vi "Plot load - plots.vi"(8 "error in (no error)":errorcluster, 10 "plots":T2[](array[typedef]), 11 "Refs":T4) -> (0 "error out":errorcluster, 3 "top array.value":T1[](array[typedef]))   [LabVIEW 2021, in "RocketPlot.lvlib"]
uses:
  RocketPlot.lvlib
  TypeDefs/Plot UI references.ctl
  Classes/RocketPlotHandle/RocketPlotHandle.lvclass
  <userlib>/bjustice/TipStripOOPanel/Classes/TipPanelHandle/TipPanelHandle.lvclass
  TypeDefs/Plot top row.ctl
  TypeDefs/plot properties V2.ctl
  TypeDefs/plot attributes V2.ctl
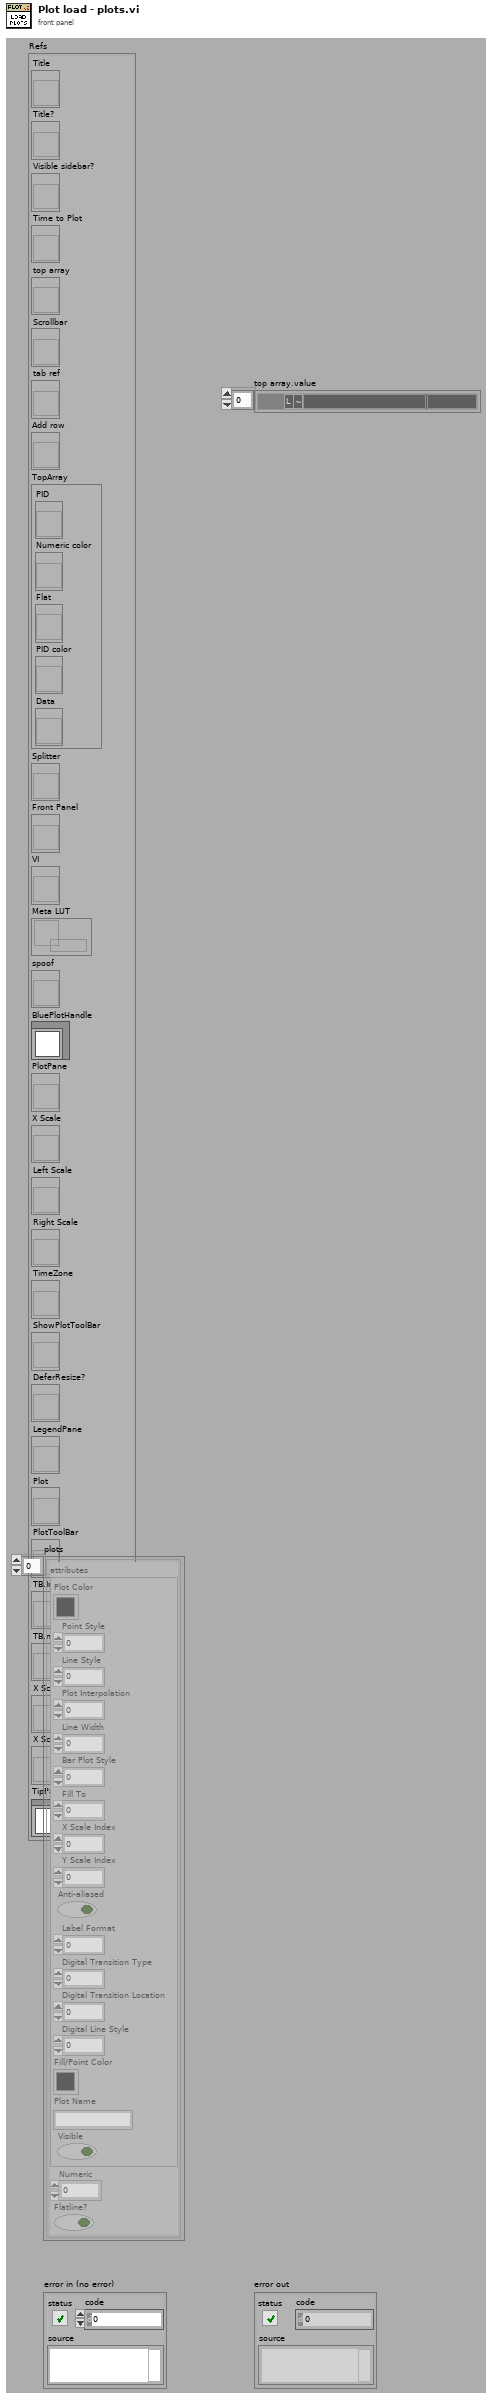
[diagram p1: front panel]
types:
  T1 = typedef "RocketPlot.lvlib/Plot top row.ctl" = cluster{"PID":string, "index":i32, "PID color":u32, "right axis?":bool, "Flatline?":bool, "Numeric color":u32, "Data":string, "Flat":string}
  T2 = typedef "RocketPlot.lvlib/plot properties V2.ctl" = cluster{"attributes":T3, "Numeric":dbl, "Flatline?":bool}
  T3 = typedef "RocketPlot.lvlib/plot attributes V2.ctl" = cluster{"Plot Color":u32, "Point Style":u8, "Line Style":u8, "Plot Interpolation":u8, "Line Width":u8, "Bar Plot Style":u8, "Fill To":i16, "X Scale Index":u32, "Y Scale Index":u32, "Anti-aliased":bool, "Label Format":u8, "Digital Transition Type":u8, "Digital Transition Location":u8, "Digital Line Style":u8, "Fill/Point Color":u32, "Plot Name":string, "Visible":bool}
  T4 = typedef "RocketPlot.lvlib/Plot UI references.ctl" = cluster{"Title":refnum<vi>, "Title?":refnum<vi>, "Visible sidebar?":refnum<vi>, "Time to Plot":refnum<vi>, "top array":refnum<vi>, "Scrollbar":refnum<vi>, "tab ref":refnum<vi>, "Add row":refnum<vi>, "TopArray":cluster{"PID":refnum<vi>, "Numeric color":refnum<vi>, "Flat":refnum<vi>, "PID color":refnum<vi>, "Data":refnum<vi>}, "Splitter":refnum<vi>, "Front Panel":refnum<vi>, "VI":refnum<vi>, "Meta LUT":refnum<data-value>, "spoof":refnum<vi>, "BluePlotHandle":refnum<class "RocketPlotHandle.lvclass">, "PlotPane":refnum<vi>, "X Scale":refnum<vi>, "Left Scale":refnum<vi>, "Right Scale":refnum<vi>, "TimeZone":refnum<vi>, "ShowPlotToolBar":refnum<vi>, "DeferResize?":refnum<vi>, "LegendPane":refnum<vi>, "Plot":refnum<vi>, "PlotToolBar":refnum<vi>, "TB.Info":refnum<vi>, "TB.max":refnum<vi>, "X Scale.Plot Name":refnum<vi>, "X Scale.Use Plot Name?":refnum<vi>, "TipPanel":refnum<class "TipPanelHandle.lvclass">}
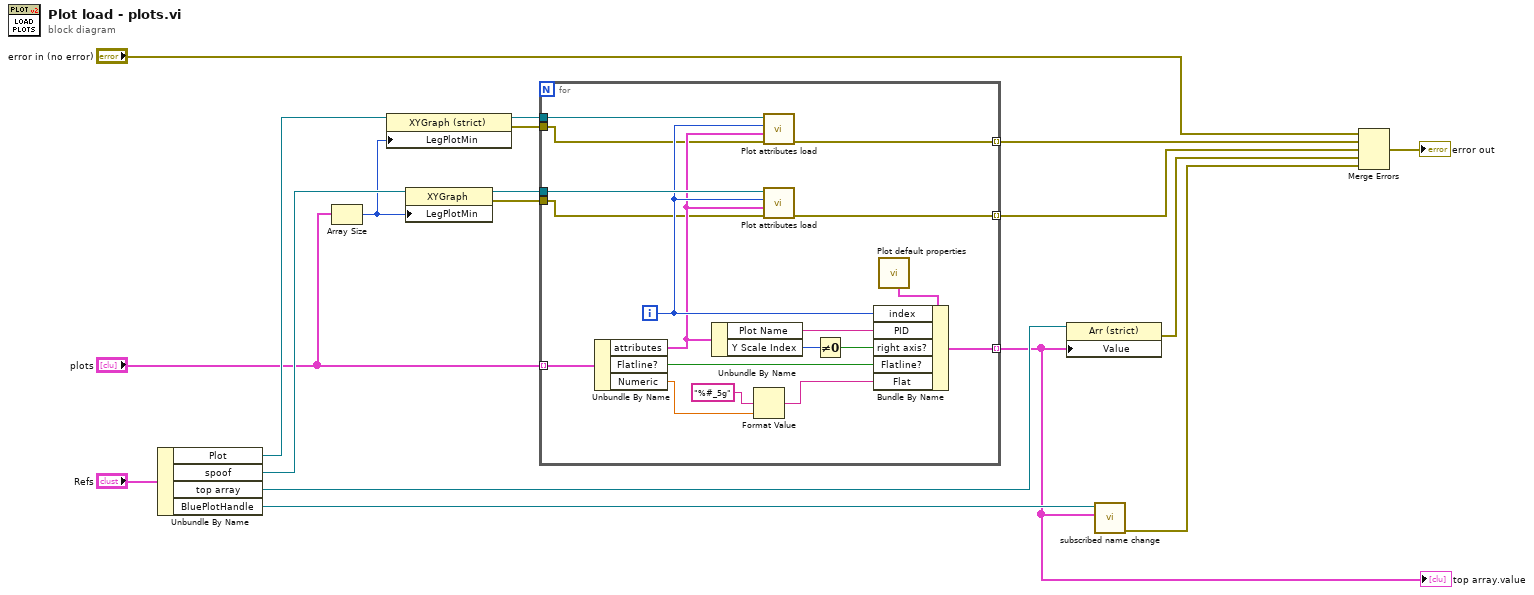
[diagram p0: block diagram]
diagram:
  n1 = Unbundle By Name("Refs") -> ("Plot"=w7:refnum<vi>, "spoof"=w13:refnum<vi>, "top array"=w18:refnum<vi>, "BluePlotHandle"=w6:refnum<class "RocketPlotHandle.lvclass">)
  n2 = Array Size(array="plots") -> (size(s)=w10:i32)
  n3 = property class="XYGraph (strict)"(reference=w7, "LegPlotMin"=w10) -> (reference out=w11:refnum<vi>, error out=w9:errorcluster)  [unwired: 1 in]
  n4 = property class="XYGraph"(reference=w13, "LegPlotMin"=w10) -> (reference out=w12:refnum<vi>, error out=w8:errorcluster)  [unwired: 1 in]
  n5 = for {
    tunnel: w11 -> [w35]
    tunnel: "plots" -> [w36] mode=indexing
    tunnel: w12 -> [w34]
    tunnel: [w27] -> w5 mode=indexing
    tunnel: [w26] -> w17 mode=indexing
    tunnel: [w25] -> w16 mode=indexing
    tunnel: w9 -> [w23]
    tunnel: w8 -> [w22]
    i -> [w33]
    n6 = Unbundle By Name(w36) -> ("attributes"=w32:T3, "Flatline?"=w28:bool, "Numeric"=w21:dbl)
    n7 = Unbundle By Name(w32) -> ("Plot Name"=w31:string, "Y Scale Index"=w30:u32)
    n8 = Format Value(format string="%#_5g", value (0)=w21) -> (output string=w19:string)  [unwired: 1 in]
    n9 = call "Plot attributes load.vi"("error in (no error)"=w23, "attributes"=w32, "Active Plot"=w33, "Plot"=w35) -> ("error out"=w26:errorcluster)  [unwired: 6 in, 1 out]
    n10 = call "Plot attributes load.vi"("error in (no error)"=w22, "attributes"=w32, "Active Plot"=w33, "Plot"=w34) -> ("error out"=w25:errorcluster)  [unwired: 6 in, 1 out]
    n11 = Not Equal To 0?(x=w30) -> (x != 0?=w29:bool)
    n12 = call "Plot default properties.vi"() -> ("Default plot UI"=w24:T1)  [unwired: 7 in, 4 out]
    n13 = Bundle By Name(cluster=w24, "index"=w33, "PID"=w31, "right axis?"=w29, "Flatline?"=w28, "Flat"=w19) -> (w27:T1)
  }
  "top array.value" <- w5
  n14 = property class="Arr (strict)"(reference=w18, "Value"=w5) -> (error out=w15:errorcluster)  [unwired: 1 in, 1 out]
  n15 = call "subscribed name change.vi"("top array"=w5, "BluePlotHandle"=w6) -> ("error out"=w4:errorcluster)  [unwired: 9 in]
  n16 = Merge Errors("error in (no error)", w17, w16, w15, w4) -> (→"error out":errorcluster)
